vi "posi incial-proceso 1.vi"() -> ()   [LabVIEW 2020]
panel:
  in  "posi-inicial proceso 1":T1
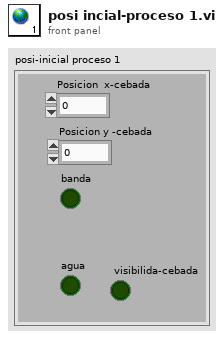
[diagram p1: front panel]
types:
  T1 = cluster{"Posicion  x-cebada":dbl, "banda":bool, "agua":bool, "Posicion y -cebada ":dbl, " visibilida-cebada":bool}
diagram:
